vi "Generate voltage.vi"(8 "error in (no error)":errorcluster, 11 "RSA in":refnum<class "RSA.lvclass">) -> (0 "error out":errorcluster, 3 "RSA out":refnum<class "RSA.lvclass">)   [LabVIEW 2012, in "RSA.lvclass"]
uses:
  RSA.lvclass
  RSA.lvclass/RSA.ctl
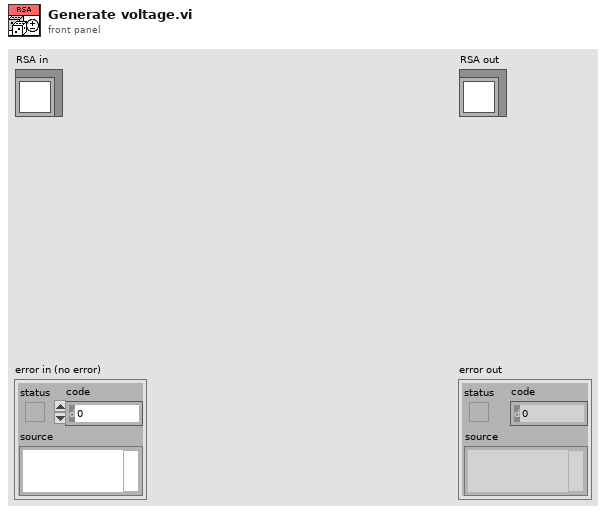
[diagram p1: front panel]
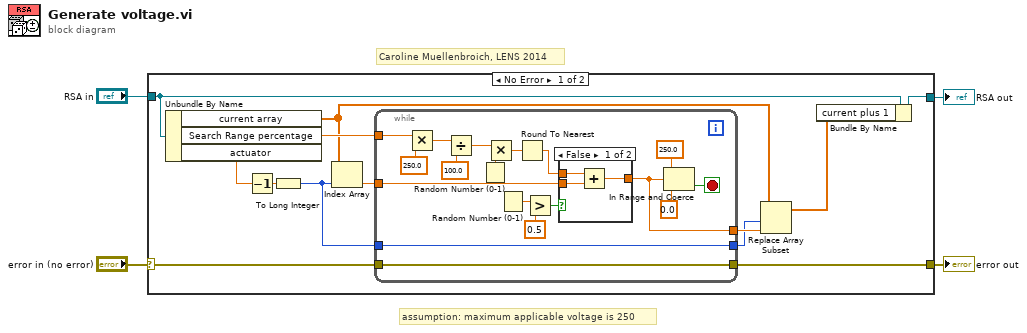
[diagram p0: block diagram]
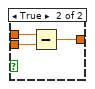
[diagram p2: hidden frame]
diagram:
  # "Caroline Muellenbroich, LENS 2014"
  # "assumption: maximum applicable voltage is 250"
  n1 = case shown="No Error" "error in (no error)" {
    selector: "error in (no error)" -> [w12 w43]
    tunnel: [w14 w43] -> w3
    tunnel: [w7 w42] -> w1
    tunnel: "RSA in" -> [w11 w42]
    frame No Error {
      n2 = Unbundle By Name(w11) -> ("current array"=w10:dbl[], "Search Range percentage"=w16:dbl, "actuator"=w5:dbl)
      n3 = Decrement(x=w5) -> (x-1=w17:dbl)
      n4 = To Long Integer(number=w17) -> (32bit integer=w13:i32)
      n5 = Index Array(array=w10, index=w13) -> (element=w15:dbl)
      n6 = while {
        tunnel: w16 -> [w35]
        tunnel: w15 -> [w25]
        tunnel: [w20] -> w9
        tunnel: w12 -> [w19]
        tunnel: [w19] -> w14
        tunnel: [w18] -> w8
        tunnel: w13 -> [w18]
        stop <- w21 stop-if-true
        n7 = Multiply(x=w35, y=250.0 ("upper limit")) -> (x*y=w33:dbl)
        n8 = Divide(x=w33, y=100.0) -> (x/y=w30:dbl)
        n9 = Random Number (0-1)() -> (number: 0 to 1=w31:dbl)
        n10 = Multiply(x=w30, y=w31) -> (x*y=w29:dbl)
        n11 = Random Number (0-1)() -> (number: 0 to 1=w28:dbl)
        n12 = Round To Nearest(number=w29) -> (nearest integer value=w24:dbl)
        n13 = Greater?(x=w28, y=0.5) -> (0:w26:bool)
        n14 = case shown="False" w26 {
          tunnel: w25 -> [w36 w39]
          tunnel: w24 -> [w38 w41]
          tunnel: [w37 w40] -> w20
          frame False {
            n15 = Add(x=w38, y=w36) -> (x+y=w37:dbl)
          }
          frame True {
            n16 = Subtract(x=w41, y=w39) -> (x-y=w40:dbl)
          }
        }
        n17 = In Range and Coerce(upper limit=250.0, x=w20, lower limit=0.0) -> (In Range?=w21:bool)  [unwired: 1 out]
      }
      n18 = Replace Array Subset(array=w10, new element=w9, index=w8) -> (w6:dbl[])
      n19 = Bundle By Name(cluster=w11, "current plus 1"=w6) -> (w7:refnum<class "RSA.lvclass">)
    }
    frame Error {
    }
  }
  "error out" <- w3
  "RSA out" <- w1
